vi "divergence.vi"() -> ()   [LabVIEW 2011]
uses:
  <userlib>/_OpenG.lib/array/array.llb/Sort 2D Array (DBL)__ogtk.vi
panel:
  out "XY Graph 4":cluster{dbl[], dbl[]}(graph)
  out "ceil(x): smallest int >= x":dbl
  out "subarray":dbl[](graph)
  out "size(s)":i32
  out "fractional index or x":dbl
  out "XY Graph 6":cluster{dbl[], dbl[]}(graph)={[nan, -22.39776866049278, -22.197753113900514, -21.99475551202534, -21.797849731203137, -21.572711439872613, -21.375999648112447, -21.175009746455803, -20.97856592300744, -20.760769615289096, -20.560330872149162, -20.35943166582951, -20.165065187036877, -19.948386526301867, -19.74215265466412, -19.54226357579135, -19.34822990149488, -19.137393946788265, -18.933444658504254, -18.737616023076534, -18.53817031412297, -18.322190487627786, -18.121740027906547, -17.925694204356624, -17.729966277380896, -17.517412864070373, -17.31348940241019, -17.11289801811939, -16.915686366945977, -16.705802533526995, -16.505712601127016, -16.30739451938342, -16.109356883288758, -15.894334110287307, -15.687578221493734, -15.494623089638345, -15.300149648385856, -15.088491177406018, -14.882546906173513, -14.683590103931857, -14.487049554247383, -14.2724196957884, -14.072672908359023, -13.876515933006377, -13.681180604820462, -13.465217116646162, -13.25976105466579, -13.06125813397039, -12.869240919662257, -12.65761281753555, -12.453137786207463, -12.255611419771016, -12.059695402232325, -11.838863864806859, -11.638805288951135, -11.447486602098714, -11.250197538257574, -11.035800171352387, -10.829738293707951, -10.633508746918208, -10.438435962702137, -10.221833280055245, -10.021724707453576, -9.826354982933028, -9.634611816673615, -9.412439543136108, -9.20511724840586, -9.008417599709512, -8.825954548325072, -8.606634690839229, -8.400333221492458, -8.20261655221582, -8.011435815272016, -7.784746585498241, -7.589688365482455, -7.395645274047141, -7.207938565651453, -6.983253325987057, -6.77575627855926, -6.578994814558614, -6.39315963291095, -6.172483288816173, -5.967815890125991, -5.777299052364459, -5.588806322459376, -5.355813323486949, -5.145358133416896, -4.964595740248905, -4.787885451800403, -4.551409317547562, -4.345249015876691, -4.153086836211923, -3.968784333391284, -3.73133965541636, -3.53031808389975, -3.3489832787216356, -3.1779597732662377, -2.926740080174682, -2.708648964839888, -2.5097985181559985, -2.3761497977844623, -2.1187265344634243, -1.9082946597117758, -1.7251354446661915, -1.5711976326752473, -1.2796887279197522, -1.0553692415378784, -0.9033280207367064, -0.79550183720515, -0.5118754911679008, -0.2559377455839503, 0.0, nan, 0.281915746402599, 0.5118754911679009, 0.7678132367518513, 1.0231123851178776, 1.037198652538229, 1.273753440093689, 1.527010646980553, 1.7908430132888096, 1.8954995279040867, 2.115134111105165, 2.3414884144252888, 2.567479231121357, 2.6882411640961434, 2.92360960275587, 3.1530911495681613, 3.381022017744267, 3.5276542514174123, 3.730087138641882, 3.9478673505586346, 4.174073236005483, 4.344242053650726, 4.550355833050645, 4.767623435089535, 4.986866048510827, 5.147809482817562, 5.348931768591219, 5.57367561426017, 5.793373223377384, 5.9686324707625005, 6.169861717253209, 6.382520257293259, 6.592777744132338, 6.774034504145342, 6.9814567592769, 7.1957717395243455, 7.408965677978099, 7.587979090470806, 7.7892452664406, 7.9951972139117125, 8.216296126538069, 8.399196524345204, 8.604919583757509, 8.815825817218652, 9.023508994511403, 9.202000866445353, 9.4108434412504, 9.624273191193655, 9.836812029917615, 10.0214043022762, 10.222685086451294, 10.429450378697583, 10.641047312920259, 10.830614719685446, 11.033811782904275, 11.24416883888916, 11.451621425407527, 11.643056613539558, 11.838761084216719, 12.04869128799522, 12.264086613205661, 12.4536188062357, 12.65611744560156, 12.863708361520652, 13.068685853458444, 13.259062006573528, 13.464187000477843, 13.673957000257655, 13.882965018738679, 14.073392676176983, 14.273531326058409, 14.478984758303463, 14.689899458558896, 14.883001045908888, 15.086529328977301, 15.295295334959823, 15.499913423595729, 15.690656481332129, 15.891150436745738, 16.11259871657597, 16.320535754147848, 16.514758182702487, 16.716155828887878, 16.92969101670736, 17.145138992923055, 17.331769007550296, 17.55012744962851, 17.722572893404024], [0.0, 0.0, 0.0, 0.0, 0.0, 0.0, 0.0, 0.0, 0.0, 0.0, 0.0, 0.0, 0.0, 0.0, 0.0, 0.0, 0.0, 0.0, 0.0, 0.0, 0.0, 0.0, 0.0, 0.0, 0.0, 0.0, 0.0, 0.0, 0.0, 0.0, 0.0, 0.0, 0.0, 0.0, 0.0, 0.0, 0.0, 0.0, 0.0, 0.0, 0.0, 0.0, 0.0, 0.0, 0.0, 0.0, 0.0, 0.0, 0.0, 0.0, 0.0, 0.0, 0.0, 0.0, 0.0, 0.0, 0.0, 0.0, 0.0, 0.0, 0.0, 0.0, 0.0, 0.0, 0.0, 0.0, 0.0, 0.0, 0.0, 0.0, 0.0, 0.0, 0.0, 0.0, 0.0, 0.0, 0.0, 0.0, 0.0, 0.0, 0.0, 0.00017512613576245854, 0.0, 0.0, 0.0, 0.0, 0.0, 0.0, 0.0, 0.0, 0.0, 0.0, 0.0, 0.0, 0.0, 0.0, 0.0, 0.0, 0.0, 0.0, 0.0, 0.0012142117787156703, 0.00841639058042327, 0.02449355095831155, 0.0, 0.06725045973578939, 0.018747820990586854, 0.11159238170527333, 0.016389792621155613, 0.19690238656338716, 0.24494044386338287, 0.2921073201597638, 0.0, 0.5625304152043127, 0.33763957239371256, 0.33762793112921285, 0.3267042392929598, 0.0, 0.03201705843741025, 0.2222956021137524, 0.2497366879861331, 0.2180346846753834, 0.1839846296823897, 0.12738716757860738, 0.05574712431823763, 0.10393790022878097, 0.058508089714605485, 0.022873596308455722, 0.0032490550557084216, 0.004163777776645822, 0.0001589989492762092, 0.00014953147131881669, 0.0, 0.00014972365572693048, 0.0, 0.0, 0.0, 0.0, 0.0, 0.0, 0.0, 0.0, 0.0, 0.0, 0.0, 0.0, 0.0, 0.0, 0.0, 0.0, 0.0, 0.0, 0.0, 0.0, 0.0, 0.0, 0.0, 0.0, 0.0, 0.0, 0.0, 0.0, 0.0, 0.0, 0.0, 0.0, 0.0, 0.0, 0.0, 0.0, 0.0, 0.0, 0.0, 0.0, 0.0, 0.0, 0.0, 0.0, 0.0, 0.0, 0.0, 0.0, 0.0, 0.0, 0.0, 0.0, 0.0, 0.0, 0.0, 0.0, 0.0, 0.0, 0.0, 0.0, 0.0, 0.0, 0.0, 0.0, 0.0, 0.0]}
  out "size(s) 2":i32
  out "Waveform Graph":i32[](graph)
  out "XY Graph 5":cluster{dbl[], dbl[]}(graph)={[nan, -22.39776866049278, -22.197753113900514, -21.99475551202534, -21.797849731203137, -21.572711439872613, -21.375999648112447, -21.175009746455803, -20.97856592300744, -20.760769615289096, -20.560330872149162, -20.35943166582951, -20.165065187036877, -19.948386526301867, -19.74215265466412, -19.54226357579135, -19.34822990149488, -19.137393946788265, -18.933444658504254, -18.737616023076534, -18.53817031412297, -18.322190487627786, -18.121740027906547, -17.925694204356624, -17.729966277380896, -17.517412864070373, -17.31348940241019, -17.11289801811939, -16.915686366945977, -16.705802533526995, -16.505712601127016, -16.30739451938342, -16.109356883288758, -15.894334110287307, -15.687578221493734, -15.494623089638345, -15.300149648385856, -15.088491177406018, -14.882546906173513, -14.683590103931857, -14.487049554247383, -14.2724196957884, -14.072672908359023, -13.876515933006377, -13.681180604820462, -13.465217116646162, -13.25976105466579, -13.06125813397039, -12.869240919662257, -12.65761281753555, -12.453137786207463, -12.255611419771016, -12.059695402232325, -11.838863864806859, -11.638805288951135, -11.447486602098714, -11.250197538257574, -11.035800171352387, -10.829738293707951, -10.633508746918208, -10.438435962702137, -10.221833280055245, -10.021724707453576, -9.826354982933028, -9.634611816673615, -9.412439543136108, -9.20511724840586, -9.008417599709512, -8.825954548325072, -8.606634690839229, -8.400333221492458, -8.20261655221582, -8.011435815272016, -7.784746585498241, -7.589688365482455, -7.395645274047141, -7.207938565651453, -6.983253325987057, -6.77575627855926, -6.578994814558614, -6.39315963291095, -6.172483288816173, -5.967815890125991, -5.777299052364459, -5.588806322459376, -5.355813323486949, -5.145358133416896, -4.964595740248905, -4.787885451800403, -4.551409317547562, -4.345249015876691, -4.153086836211923, -3.968784333391284, -3.73133965541636, -3.53031808389975, -3.3489832787216356, -3.1779597732662377, -2.926740080174682, -2.708648964839888, -2.5097985181559985, -2.3761497977844623, -2.1187265344634243, -1.9082946597117758, -1.7251354446661915, -1.5711976326752473, -1.2796887279197522, -1.0553692415378784, -0.9033280207367064, -0.79550183720515, -0.5118754911679008, -0.2559377455839503, 0.0, nan, 0.281915746402599, 0.5118754911679009, 0.7678132367518513, 1.0231123851178776, 1.037198652538229, 1.273753440093689, 1.527010646980553, 1.7908430132888096, 1.8954995279040867, 2.115134111105165, 2.3414884144252888, 2.567479231121357, 2.6882411640961434, 2.92360960275587, 3.1530911495681613, 3.381022017744267, 3.5276542514174123, 3.730087138641882, 3.9478673505586346, 4.174073236005483, 4.344242053650726, 4.550355833050645, 4.767623435089535, 4.986866048510827, 5.147809482817562, 5.348931768591219, 5.57367561426017, 5.793373223377384, 5.9686324707625005, 6.169861717253209, 6.382520257293259, 6.592777744132338, 6.774034504145342, 6.9814567592769, 7.1957717395243455, 7.408965677978099, 7.587979090470806, 7.7892452664406, 7.9951972139117125, 8.216296126538069, 8.399196524345204, 8.604919583757509, 8.815825817218652, 9.023508994511403, 9.202000866445353, 9.4108434412504, 9.624273191193655, 9.836812029917615, 10.0214043022762, 10.222685086451294, 10.429450378697583, 10.641047312920259, 10.830614719685446, 11.033811782904275, 11.24416883888916, 11.451621425407527, 11.643056613539558, 11.838761084216719, 12.04869128799522, 12.264086613205661, 12.4536188062357, 12.65611744560156, 12.863708361520652, 13.068685853458444, 13.259062006573528, 13.464187000477843, 13.673957000257655, 13.882965018738679, 14.073392676176983, 14.273531326058409, 14.478984758303463, 14.689899458558896, 14.883001045908888, 15.086529328977301, 15.295295334959823, 15.499913423595729, 15.690656481332129, 15.891150436745738, 16.11259871657597, 16.320535754147848, 16.514758182702487, 16.716155828887878, 16.92969101670736, 17.145138992923055, 17.331769007550296, 17.55012744962851, 17.722572893404024], [0.0, 0.0, 0.0, 0.0, 0.0, 0.0, 0.0, 0.0, 0.0, 0.0, 0.0, 0.0, 0.0, 0.0, 0.0, 0.0, 0.0, 0.0, 0.0, 0.0, 0.0, 0.0, 0.0, 0.0, 0.0, 0.0, 0.0, 0.0, 0.0, 0.0, 0.0, 0.0, 0.0, 0.0, 0.0, 0.0, 0.0, 0.0, 0.0, 0.0, 0.0, 0.0, 0.0, 0.0, 0.0, 0.0, 0.0, 0.0, 0.0, 0.0, 0.0, 0.0, 0.0, 0.0, 0.0, 0.0, 0.0, 0.0, 0.0, 0.0, 0.0, 0.0, 0.0, 0.0, 0.0, 0.0, 0.0, 0.0, 0.0, 0.0, 0.0, 0.0, 0.0, 0.0, 0.0, 0.0, 0.0, 0.0, 0.0, 0.0, 0.0, 0.00017512613576245854, 0.0, 0.0, 0.0, 0.0, 0.0, 0.0, 0.0, 0.0, 0.0, 0.0, 0.0, 0.0, 0.0, 0.0, 0.0, 0.0, 0.0, 0.0, 0.0, 0.0012142117787156703, 0.00841639058042327, 0.02449355095831155, 0.0, 0.06725045973578939, 0.018747820990586854, 0.11159238170527333, 0.016389792621155613, 0.19690238656338716, 0.24494044386338287, 0.2921073201597638, 0.0, 0.5625304152043127, 0.33763957239371256, 0.33762793112921285, 0.3267042392929598, 0.0, 0.03201705843741025, 0.2222956021137524, 0.2497366879861331, 0.2180346846753834, 0.1839846296823897, 0.12738716757860738, 0.05574712431823763, 0.10393790022878097, 0.058508089714605485, 0.022873596308455722, 0.0032490550557084216, 0.004163777776645822, 0.0001589989492762092, 0.00014953147131881669, 0.0, 0.00014972365572693048, 0.0, 0.0, 0.0, 0.0, 0.0, 0.0, 0.0, 0.0, 0.0, 0.0, 0.0, 0.0, 0.0, 0.0, 0.0, 0.0, 0.0, 0.0, 0.0, 0.0, 0.0, 0.0, 0.0, 0.0, 0.0, 0.0, 0.0, 0.0, 0.0, 0.0, 0.0, 0.0, 0.0, 0.0, 0.0, 0.0, 0.0, 0.0, 0.0, 0.0, 0.0, 0.0, 0.0, 0.0, 0.0, 0.0, 0.0, 0.0, 0.0, 0.0, 0.0, 0.0, 0.0, 0.0, 0.0, 0.0, 0.0, 0.0, 0.0, 0.0, 0.0, 0.0, 0.0, 0.0, 0.0, 0.0]}
  in  "output array 4":dbl[](array[numeric])=array[46592 elements]
  in  "output array 3":dbl[](array[numeric])=array[46592 elements]
  out "XY Graph 3":T1(graph)
  in  "output array 2":dbl[](array[numeric])=array[77312 elements]
  in  "output array":dbl[](array[numeric])=array[77312 elements]
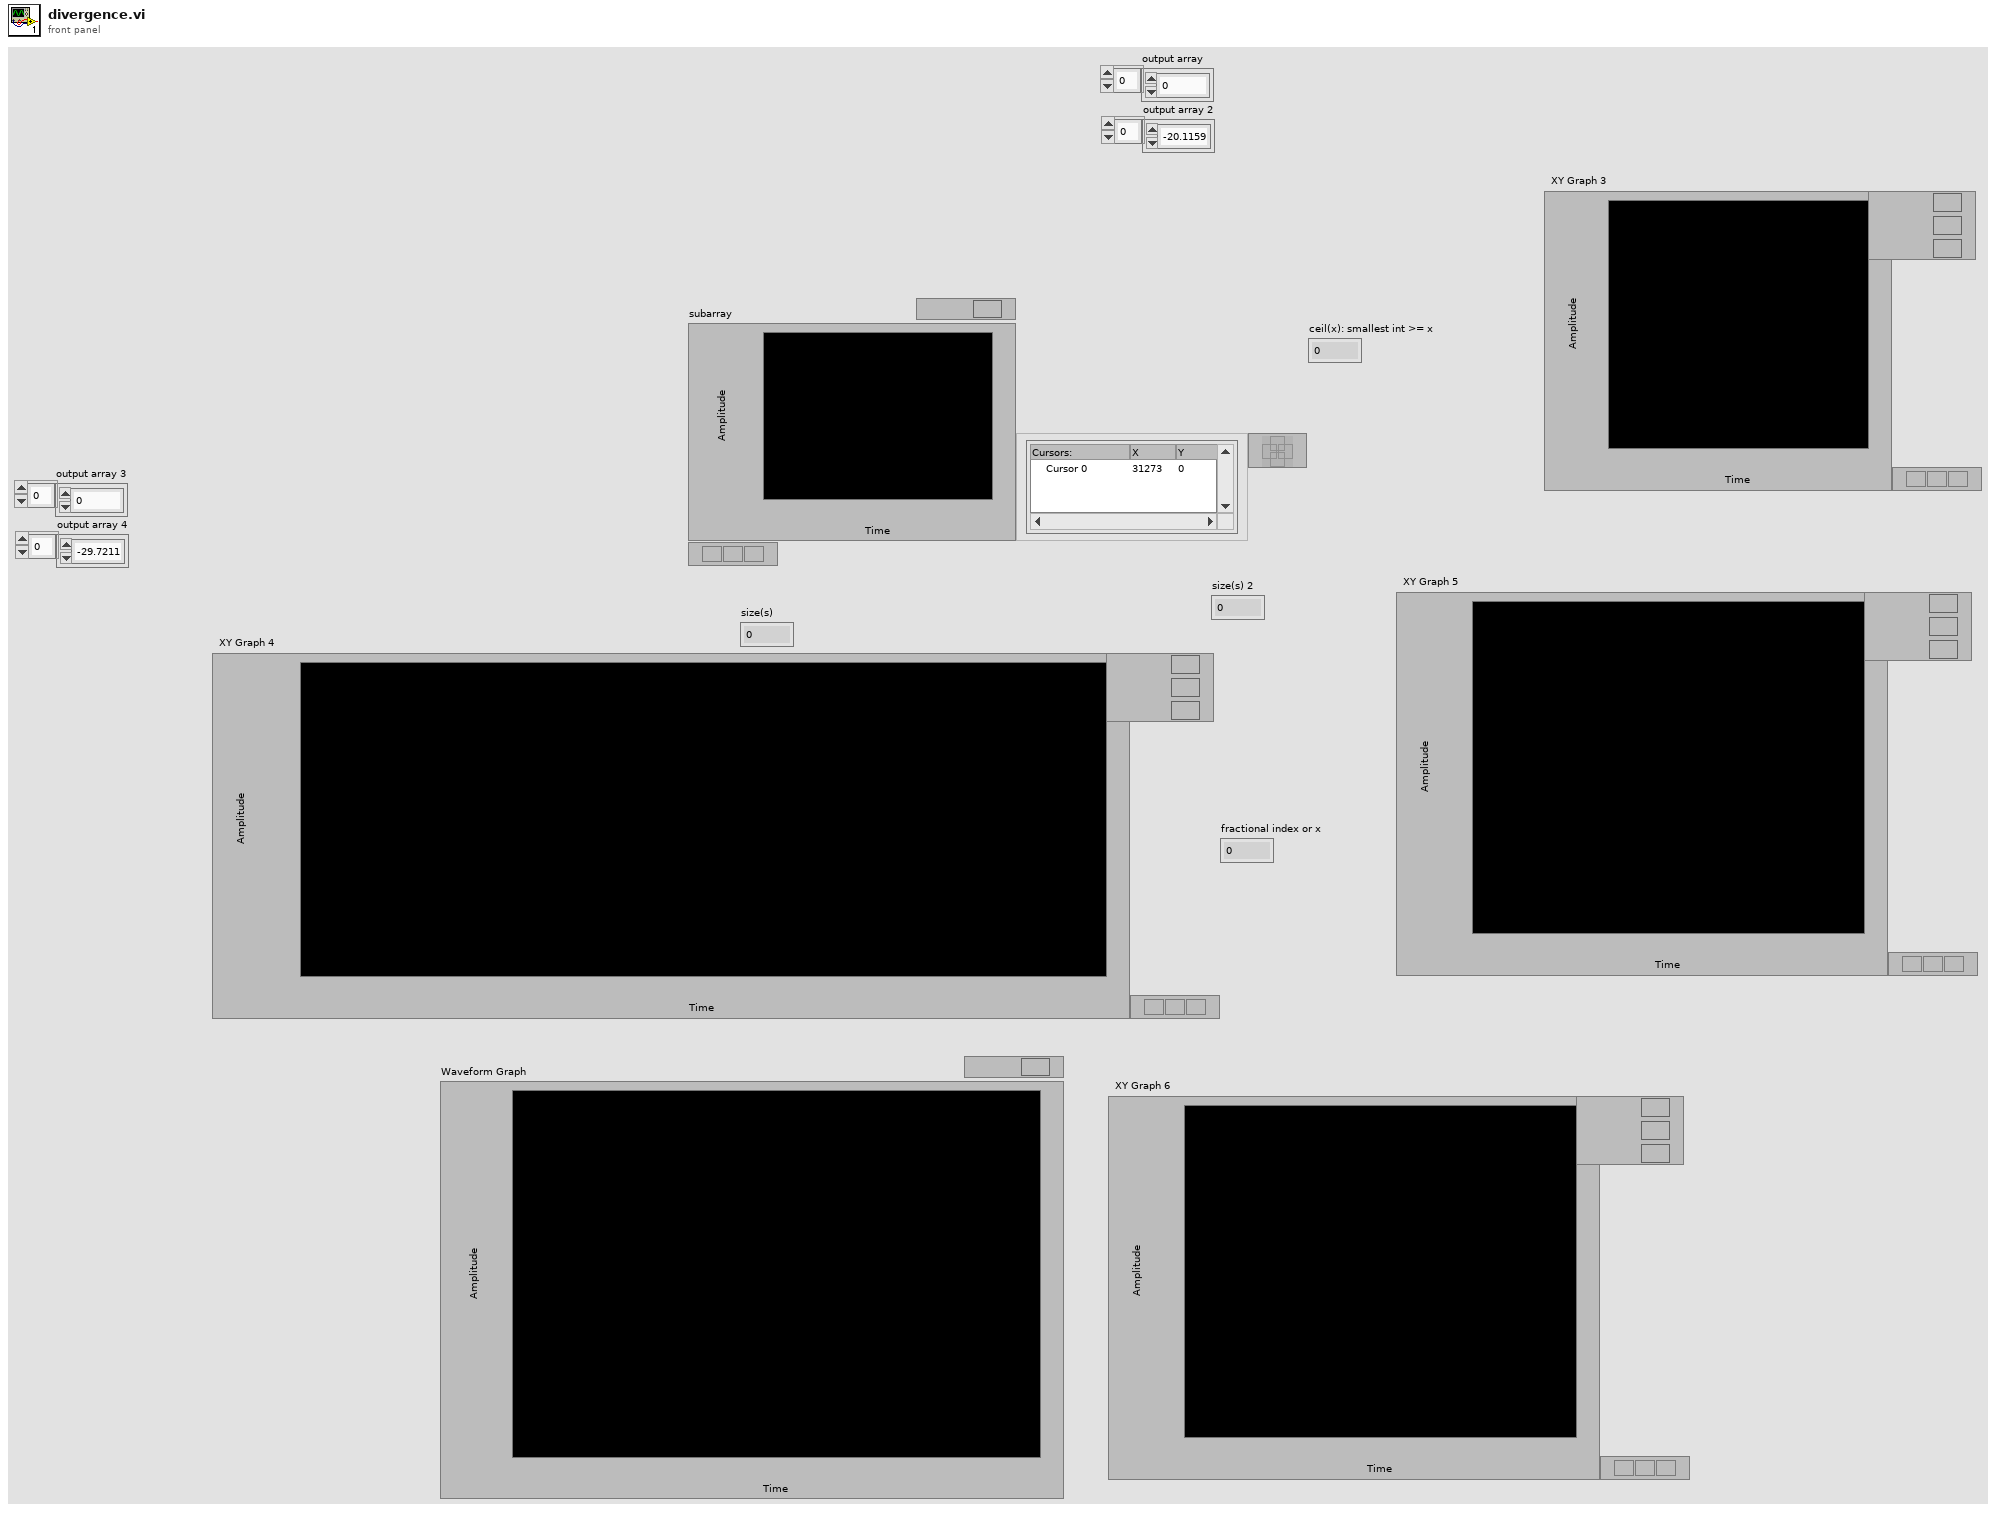
[diagram p1: front panel]
types:
  T1 = cluster{"output array 2":dbl[], "output array":dbl[]}[]
  T2 = cluster{"Sorted Array out":dbl[], "Sorted Array out":dbl[]}
  T3 = cluster{"output array 2":dbl[], "output array":dbl[]}
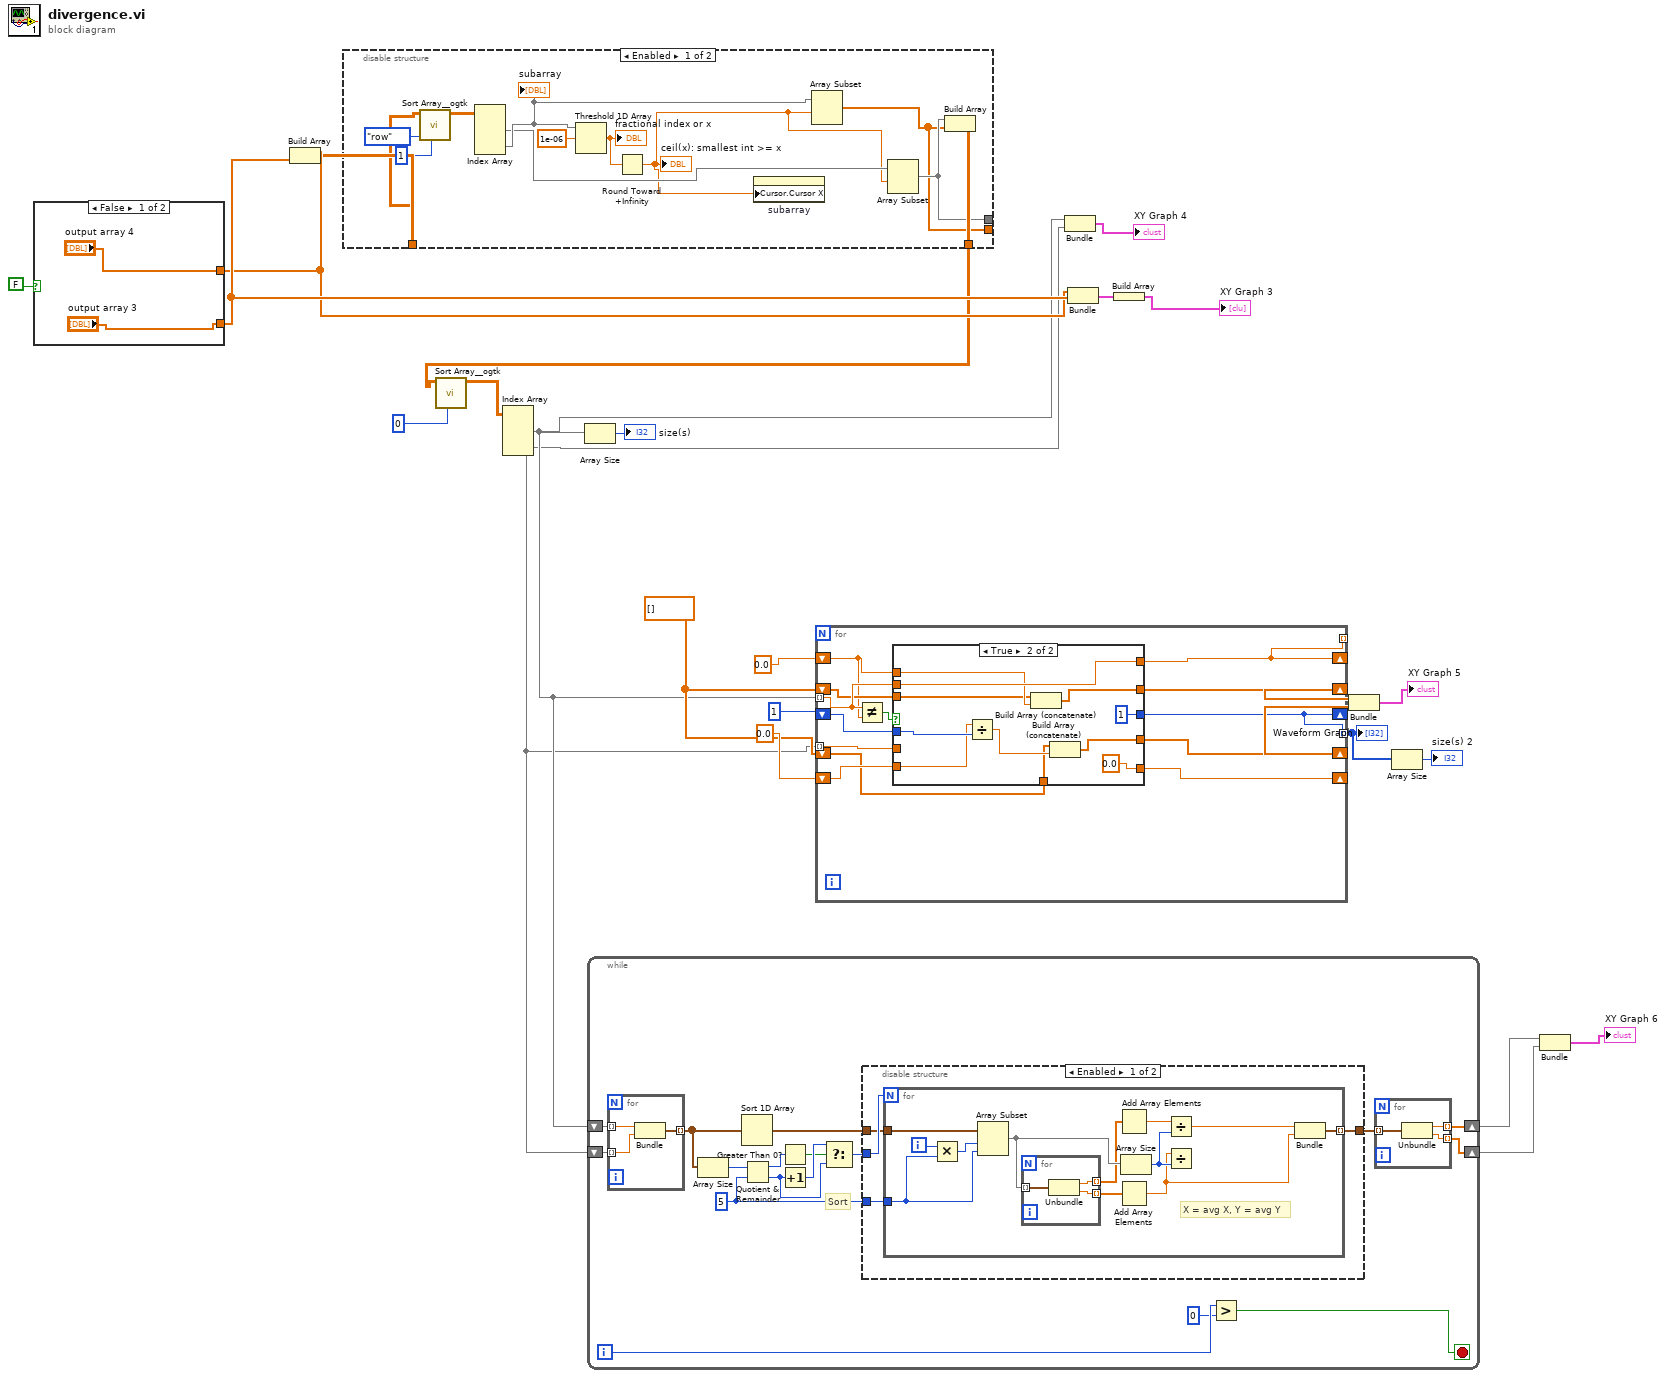
[diagram p0: block diagram]
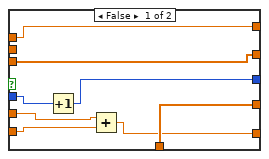
[diagram p4: hidden frame]
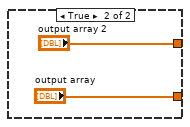
[diagram p5: hidden frame]
diagram:
  w15 = dbl[] []
  n1 = case shown="False" FALSE {
    tunnel: ["output array 3" "output array"] -> w21
    tunnel: ["output array 4" "output array 2"] -> w20
    frame False {
    }
    frame True {
    }
  }
  n2 = Build Array(w20, w21) -> (w6:dbl[][])
  n3 = disable-structure shown="Enabled" {
    disable-tunnel: w6 -> [w37 _]
    disable-tunnel: [w32 _] -> w4
    disable-tunnel: [w31 _] -> _
    disable-tunnel: [w30 _] -> _
    frame Enabled {
      n4 = call-poly <userlib>:"Sort Array__ogtk.vi"("Column/Row to Sort By"=u32 1, "Sort By in"=enum16{"row", "column"}."row", "Array in"=w37) -> ("Sorted Array out"=w40:dbl[][])  [unwired: 5 in, 3 out]
      n5 = Index Array(array=w40) -> (element #1=w34:dbl[], element #2=w35:dbl[])  [unwired: 4 in]
      "subarray" <- w35
      n6 = Threshold 1D Array(2:1e-06 ("threshold y"), 3:w35) -> (0:w38:dbl)  [unwired: 1 in]
      "fractional index or x" <- w38
      n7 = Round Toward +Infinity(x=w38) -> (ceil(x): smallest int >= x=w33:dbl)
      "ceil(x): smallest int >= x" <- w33
      n8 = property on="subarray" class="WFGraph (strict)"("Cursor.Cursor X"=w33) -> ()  [unwired: 2 in, 2 out]
      n9 = Array Subset(array=w35, index=w33) -> (w30:dbl[])  [unwired: 1 in]
      n10 = Array Subset(array=w34, index=w33) -> (w31:dbl[])  [unwired: 1 in]
      n11 = Build Array(w31, w30) -> (w32:dbl[][])
    }
    frame Disabled {
    }
  }
  n12 = call-poly <userlib>:"Sort Array__ogtk.vi"("Column/Row to Sort By"=u32 0, "Array in"=w4) -> ("Sorted Array out"=w22:dbl[][])  [unwired: 6 in, 3 out]
  n13 = Index Array(array=w22) -> (element #1=w2:dbl[], element #2=w1:dbl[])  [unwired: 4 in]
  n14 = Array Size(array=w2) -> (size(s)=→"size(s)":i32)
  n15 = while {
    shift-right: [w46] -> w9
    shift-left: w2 -> [w48]
    shift-right: [w45] -> w8
    shift-left: w1 -> [w47]
    i -> [w44]
    stop <- w43 stop-if-true
    w54 = 5 ("Samples/bin")
    # "Sort"
    n16 = for {
      tunnel: w48 -> [w84] mode=indexing
      tunnel: w47 -> [w83] mode=indexing
      tunnel: [w82] -> w51 mode=indexing
      n17 = Bundle("Numeric"=w84, "Numeric"=w83) -> (w82:cluster{"Numeric":dbl, "Numeric":dbl})  [unwired: 1 in]
    }
    n18 = Array Size(array=w51) -> (size(s)=w52:i32)
    n19 = Sort 1D Array(array=w51) -> (sorted array=w49:cluster{"Numeric":dbl, "Numeric":dbl}[])
    n20 = Quotient & Remainder(x=w52, y=w54) -> (x-y*floor(x/y)=w58:i32, floor(x/y)=w56:i32)
    n21 = Greater Than 0?(x=w58) -> (x > 0?=w55:bool)
    n22 = Increment(x=w56) -> (x+1=w57:i32)
    n23 = Select(t=w57, s=w55, f=w56) -> (s? t:f=w53:i32)
    n24 = disable-structure shown="Enabled" {
      disable-tunnel: w54 -> [w62 _]
      disable-tunnel: w53 -> [w61 _]
      disable-tunnel: [w60 w78] -> w50
      disable-tunnel: w49 -> [w59 w78]
      frame Enabled {
        n25 = for {
          N: w61 -> [_]
          tunnel: w59 -> [w74]
          tunnel: w62 -> [w72]
          tunnel: [w69] -> w60 mode=indexing
          i -> [w73]
          # "X = avg X, Y = avg Y"
          n26 = Multiply(x=w73, y=w72) -> (x*y=w71:i32)
          n27 = Array Subset(array=w74, index=w71, length=w72) -> (w70:cluster{"Numeric":dbl, "Numeric":dbl}[])
          n28 = for {
            tunnel: w70 -> [w77] mode=indexing
            tunnel: [w76] -> w68 mode=indexing
            tunnel: [w75] -> w67 mode=indexing
            n29 = Unbundle(w77) -> ("Numeric"=w76:dbl, "Numeric"=w75:dbl)
          }
          n30 = Add Array Elements(numeric array=w68) -> (sum=w66:dbl)
          n31 = Add Array Elements(numeric array=w67) -> (sum=w63:dbl)
          n32 = Array Size(array=w70) -> (size(s)=w65:i32)
          n33 = Divide(x=w66, y=w65) -> (x/y=w64:dbl)
          n34 = Divide(x=w63, y=w65) -> ()  [unwired: 1 out]
          n35 = Bundle(w64, "Numeric"=w63) -> (w69:cluster{dbl, "Numeric":dbl})  [unwired: 1 in]
        }
      }
      frame Disabled {
      }
    }
    n36 = Greater?(x=w44, y=0) -> (0:w43:bool)
    n37 = for {
      tunnel: w50 -> [w81] mode=indexing
      tunnel: [w80] -> w46 mode=indexing
      tunnel: [w79] -> w45 mode=indexing
      n38 = Unbundle(w81) -> (w80:dbl, "Numeric"=w79:dbl)
    }
  }
  n39 = for {
    tunnel: w2 -> [w93] mode=indexing
    tunnel: w1 -> [w97] mode=indexing
    shift-right: [w86] -> _
    shift-left: 0.0 -> [w87]
    shift-right: [w85] -> _
    shift-left: 1 -> [w94]
    shift-right: [w88] -> _
    shift-left: 0.0 -> [w95]
    shift-right: [w96] -> w14
    shift-left: w15 -> [w92]
    shift-right: [w90] -> w13
    shift-left: w15 -> [w91]
    tunnel: [w86] -> _ mode=indexing
    tunnel: [w85] -> w11 mode=indexing
    n40 = Not Equal?(x=w93, y=w87) -> (x != y?=w89:bool)
    n41 = case shown="True" w89 {
      tunnel: w97 -> [w100 _]
      tunnel: w87 -> [w105 w113]
      tunnel: [w103 w112] -> w96
      tunnel: w95 -> [w99 w115]
      tunnel: w94 -> [w102 w116]
      tunnel: [w105 w114] -> w86
      tunnel: w93 -> [_ w114]
      tunnel: w92 -> [w103 w111]
      tunnel: w91 -> [w104 w109]
      tunnel: [w104 w108] -> w90
      tunnel: [w101 1] -> w85
      tunnel: [w98 0.0] -> w88
      frame False {
        n42 = Increment(x=w102) -> (x+1=w101:i32)
        n43 = Add(x=w100, y=w99) -> (x+y=w98:dbl)
      }
      frame True {
        n44 = Divide(x=w115, y=w116) -> (x/y=w110:dbl)
        n45 = Build Array (concatenate)(w111, w113) -> (w112:dbl[])
        n46 = Build Array (concatenate)(w109, w110) -> (w108:dbl[])
      }
    }
  }
  "Waveform Graph" <- w11
  n47 = Bundle("Sorted Array out"=w2, "Sorted Array out"=w1) -> (→"XY Graph 4":T2)  [unwired: 1 in]
  n48 = Bundle("output array 2"=w20, "output array"=w21) -> (w25:T3)  [unwired: 1 in]
  n49 = Build Array(w25) -> (→"XY Graph 3":T1)
  n50 = Bundle(w14, w13) -> (→"XY Graph 5":cluster{dbl[], dbl[]})  [unwired: 1 in]
  n51 = Array Size(array=w11) -> (size(s)=→"size(s) 2":i32)
  n52 = Bundle("Sorted Array out"=w9, "Sorted Array out"=w8) -> (→"XY Graph 6":T2)  [unwired: 1 in]
